vi "Parameter Array to String.vi"(10 "Parameter Values":dbl[](array[numeric]), 11 "Parameter Labels":string[](array[string])) -> (2 "Parameter Array":cluster{"String":string, "Numeric":dbl}[](array[cluster]), 3 "Parameter String":string)   [LabVIEW 2020, in "SQSnobFit Control Panel.lvlib"]
uses:
  SQSnobFit Control Panel.lvlib
  Typedefs/Parameter.ctl
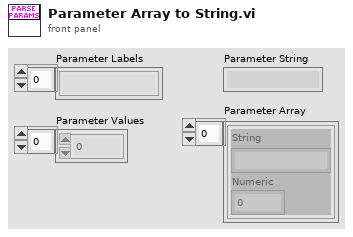
[diagram p1: front panel]
types:
  T1 = typedef "SQSnobFit Control Panel.lvlib/Parameter.ctl" = cluster{"Name":string, "Value":dbl}
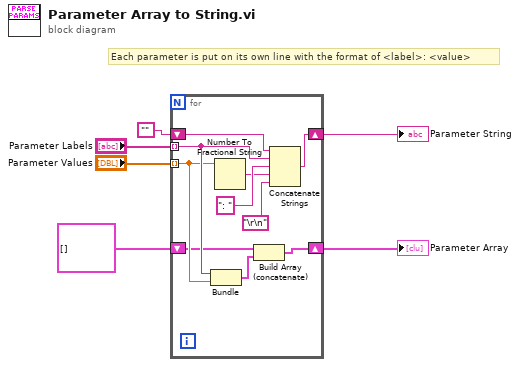
[diagram p0: block diagram]
diagram:
  # "Each parameter is put on its own line with the format of <label>: <value>"
  n1 = for {
    tunnel: "Parameter Values" -> [w10] mode=indexing
    tunnel: "Parameter Labels" -> [w11] mode=indexing
    shift-right: [w15] -> w4
    shift-left: "" -> [w14]
    shift-right: [w7] -> w1
    shift-left: T1[] [] -> [w9]
    n2 = Bundle("String"=w11, "Numeric"=w10) -> (w8:cluster{"String":string, "Numeric":dbl})  [unwired: 1 in]
    n3 = Number To Fractional String(number=w10) -> (F-format string=w12:string)  [unwired: 3 in]
    n4 = Build Array (concatenate)(w9, w8) -> (w7:T1[])
    n5 = Concatenate Strings(w14, w11, ": ", w12, "\r\n") -> (w15:string)
  }
  "Parameter String" <- w4
  "Parameter Array" <- w1
